vi "PV Clean Up Data.vi"(11 "PV Data in":string[][](array[string])) -> (3 "PV Data out":string[][](array[string]))   [LabVIEW 2023]
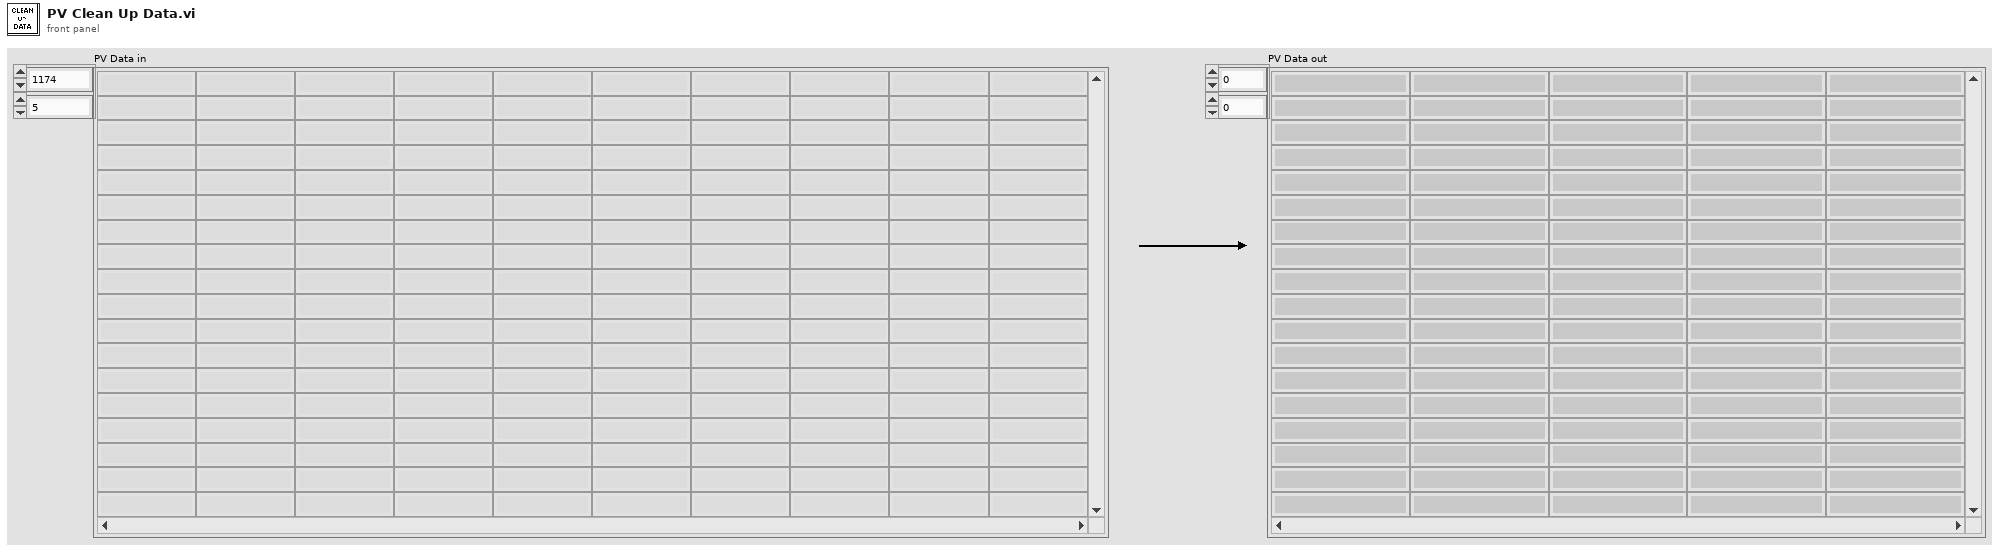
[diagram p1: front panel]
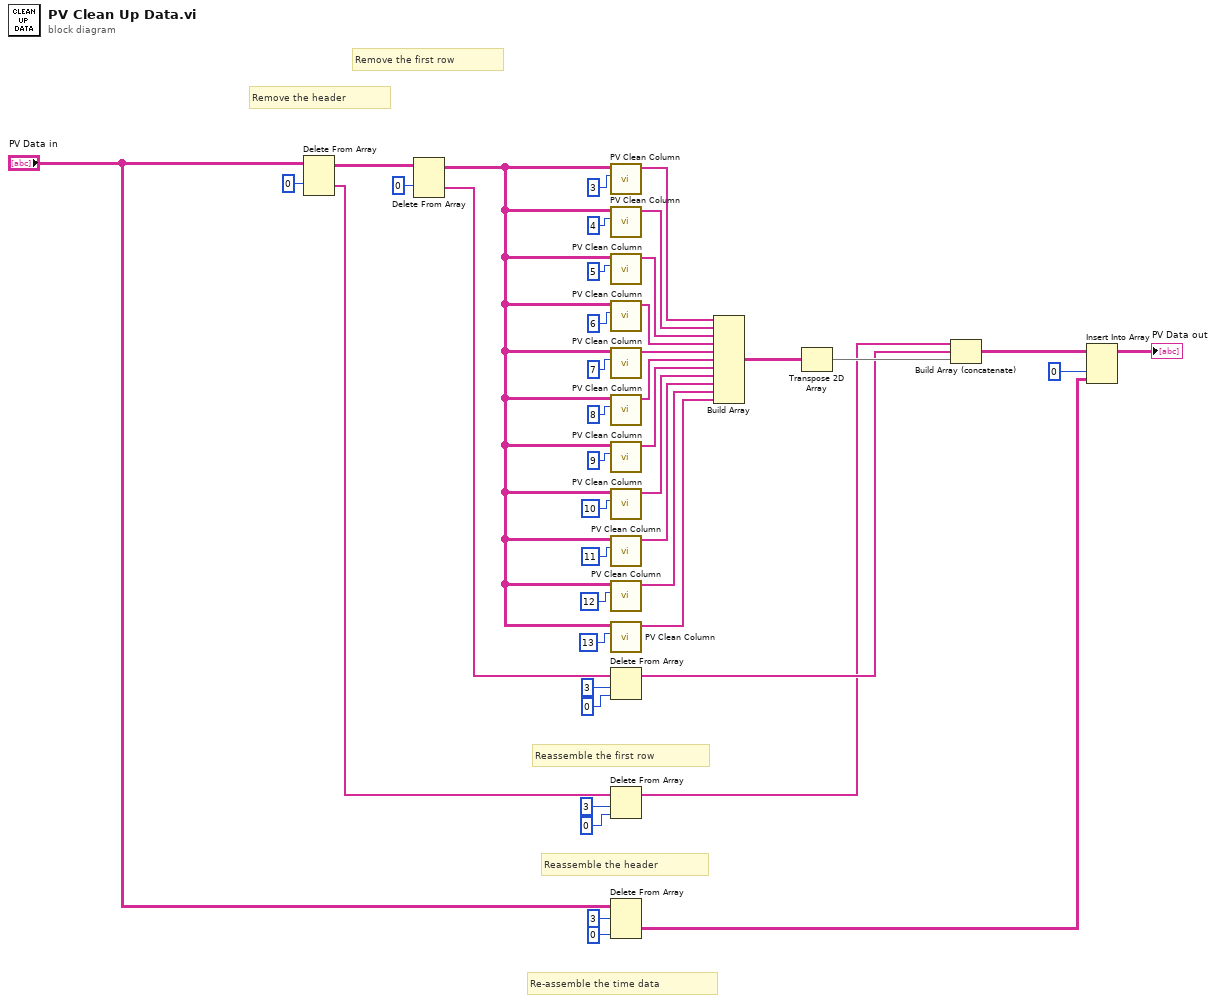
[diagram p0: block diagram]
diagram:
  # "Reassemble the first row"
  # "Reassemble the header"
  # "Re-assemble the time data"
  # "Remove the first row"
  # "Remove the header"
  n1 = Delete From Array(array="PV Data in", index (row)=0) -> (deleted portion=w20:string[], array with subset deleted=w41:string[][])  [unwired: 2 in]
  n2 = Delete From Array(array=w41, index (row)=0) -> (deleted portion=w21:string[], array with subset deleted=w3:string[][])  [unwired: 2 in]
  n3 = call "PV Clean Column.vi"("Column Number"=3, "PV Data in"=w3) -> ("Clean PV Array"=w31:string[])  [unwired: 9 in]
  n4 = call "PV Clean Column.vi"("Column Number"=4, "PV Data in"=w3) -> ("Clean PV Array"=w30:string[])  [unwired: 9 in]
  n5 = call "PV Clean Column.vi"("Column Number"=5, "PV Data in"=w3) -> ("Clean PV Array"=w29:string[])  [unwired: 9 in]
  n6 = call "PV Clean Column.vi"("Column Number"=6, "PV Data in"=w3) -> ("Clean PV Array"=w28:string[])  [unwired: 9 in]
  n7 = call "PV Clean Column.vi"("Column Number"=7, "PV Data in"=w3) -> ("Clean PV Array"=w27:string[])  [unwired: 9 in]
  n8 = call "PV Clean Column.vi"("Column Number"=8, "PV Data in"=w3) -> ("Clean PV Array"=w26:string[])  [unwired: 9 in]
  n9 = call "PV Clean Column.vi"("Column Number"=9, "PV Data in"=w3) -> ("Clean PV Array"=w25:string[])  [unwired: 9 in]
  n10 = call "PV Clean Column.vi"("Column Number"=10, "PV Data in"=w3) -> ("Clean PV Array"=w24:string[])  [unwired: 9 in]
  n11 = call "PV Clean Column.vi"("Column Number"=11, "PV Data in"=w3) -> ("Clean PV Array"=w23:string[])  [unwired: 9 in]
  n12 = call "PV Clean Column.vi"("Column Number"=12, "PV Data in"=w3) -> ("Clean PV Array"=w2:string[])  [unwired: 9 in]
  n13 = call "PV Clean Column.vi"("Column Number"=13, "PV Data in"=w3) -> ("Clean PV Array"=w1:string[])  [unwired: 9 in]
  n14 = Delete From Array(array=w21, length=3, index=0) -> (array with subset deleted=w14:string[])  [unwired: 1 out]
  n15 = Delete From Array(array=w20, length=3, index=0) -> (array with subset deleted=w13:string[])  [unwired: 1 out]
  n16 = Delete From Array(array="PV Data in", length=3, index (col)=0 ("disabled index (col)")) -> (deleted portion=w7:string[][])  [unwired: 1 in, 1 out]
  n17 = Build Array(w31, w30, w29, w28, w27, w26, w25, w24, w23, w2, w1) -> (w22:string[][])
  n18 = Transpose 2D Array(2D array=w22) -> (transposed array=w15:string[][])
  n19 = Build Array (concatenate)(w13, w14, w15) -> (w9:string[][])
  n20 = Insert Into Array(array=w9, index (col)=0 ("disabled index (col)"), new element=w7) -> (→"PV Data out":string[][])  [unwired: 1 in]
